vi "loadOceanOpticsOutputFile.vi"(11 "File":path) -> (1 "IntegrationTime":i32, 2 "Counts":dbl[](array[numeric]), 3 "wavelengths":dbl[](array[numeric]))   [LabVIEW 2011]
uses:
  <vilib>/regexp/Match Regular Expression.xnode
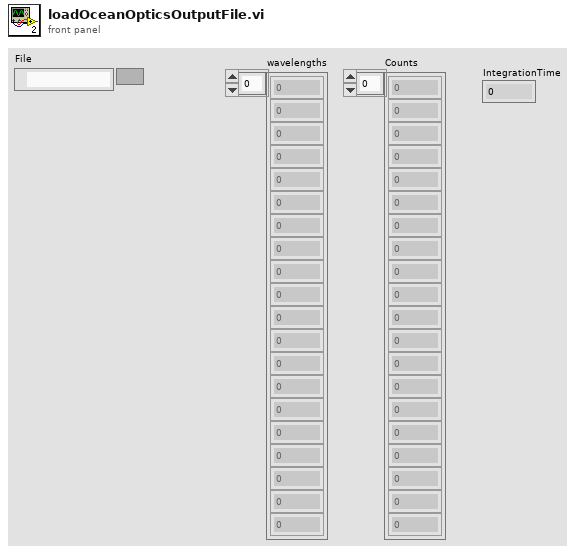
[diagram p1: front panel]
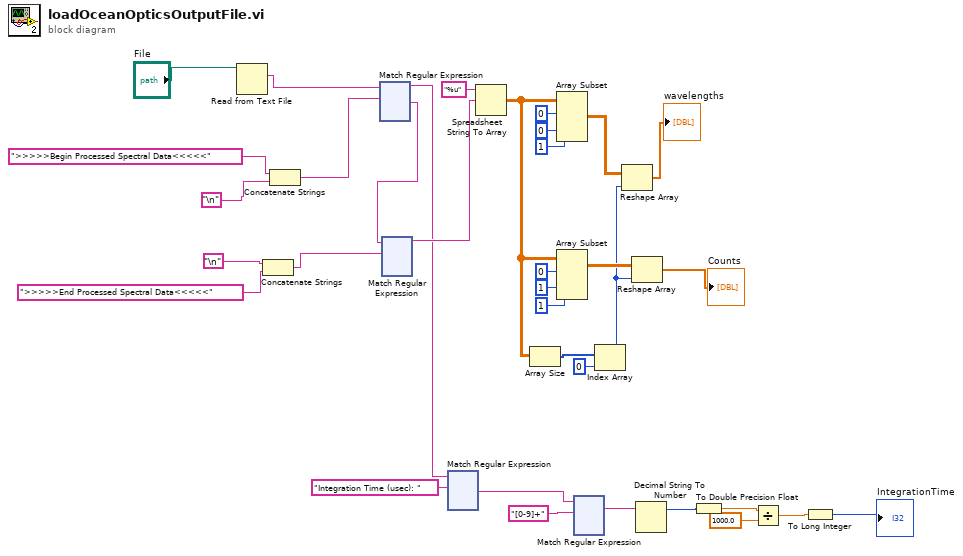
[diagram p0: block diagram]
diagram:
  n1 = Read from Text File(file (use dialog)="File") -> (text=w34:string)  [unwired: 3 in, 3 out]
  n2 = Concatenate Strings("\n", ">>>>>End Processed Spectral Data<<<<<" ("string")) -> (w11:string)
  n3 = Concatenate Strings(">>>>>Begin Processed Spectral Data<<<<<" ("regular expression"), "\n") -> (w17:string)
  n4 = xnode "Match Regular Expression"("input string"=w34, "regular expression"=w17) -> ("before match"=w10:string, "after match"=w15:string)  [unwired: 4 in, 3 out]
  n5 = xnode "Match Regular Expression"("input string"=w15, "regular expression"=w11) -> ("before match"=w14:string)  [unwired: 4 in, 4 out]
  n6 = xnode "Match Regular Expression"("input string"=w10, "regular expression"="Integration Time (usec): ") -> ("after match"=w7:string)  [unwired: 4 in, 4 out]
  n7 = Spreadsheet String To Array(format string="%u", spreadsheet string=w14) -> (array=w19:dbl[][])  [unwired: 2 in]
  n8 = Array Size(array=w19) -> (size(s)=w28:i32[])
  n9 = Array Subset(array=w19, index (row)=0 ("index"), index (col)=0 ("index"), length (col)=1 ("length")) -> (w32:dbl[][])  [unwired: 1 in]
  n10 = Array Subset(array=w19, index (row)=0 ("index"), index (col)=1 ("index"), length (col)=1 ("length")) -> (w30:dbl[][])  [unwired: 1 in]
  n11 = xnode "Match Regular Expression"("input string"=w7, "regular expression"="[0-9]+") -> ("whole match"=w6:string)  [unwired: 4 in, 4 out]
  n12 = Index Array(array=w28, index=0) -> (element=w26:i32)
  n13 = Reshape Array(w32, w26) -> (→"wavelengths":dbl[])
  n14 = Reshape Array(w30, w26) -> (→"Counts":dbl[])
  n15 = Decimal String To Number(string=w6) -> (offset past number=w3:i32)  [unwired: 2 in, 1 out]
  n16 = To Double Precision Float(number=w3) -> (double precision float=w2:dbl)
  n17 = Divide(x=w2, y=1000.0) -> (x/y=w5:dbl)
  n18 = To Long Integer(number=w5) -> (32bit integer=→"IntegrationTime":i32)
